vi "Load Config.vi"(8 "error in (no error)":errorcluster, 11 "Data Processor Module in":refnum<class "Data Processor Module.lvclass">) -> (0 "error out":errorcluster, 3 "Data Processor Module out":refnum<class "Data Processor Module.lvclass">)   [LabVIEW 2020, in "VolatusData.lvlib" / "Data Processor Module.lvclass"]
uses:
  Data Processor Module.lvclass
  Data Processor Module.lvclass/Data Processor Module.ctl
  Volatus/Module/Module.lvclass
  VolatusConfig/VolatusConfigElement/VolatusConfigElement.lvclass
  lv-cdm/CDM-Config/Config Element/Config Element.lvclass
  C:/dev/lv20CE/relink/lv-volatus/Volatus/Module/Module.lvclass
  C:/dev/lv20CE/relink/lv-volatus/VolatusData/Data Processor Module/Data Processor Module.lvclass
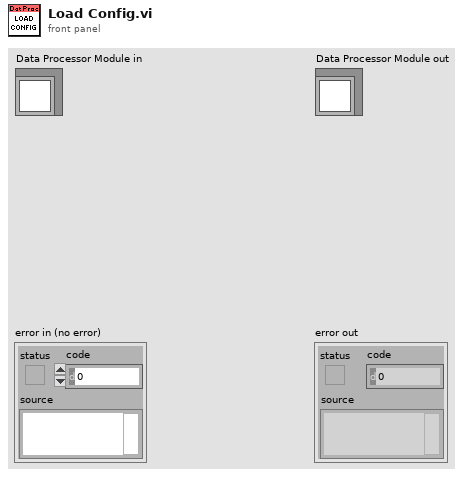
[diagram p1: front panel]
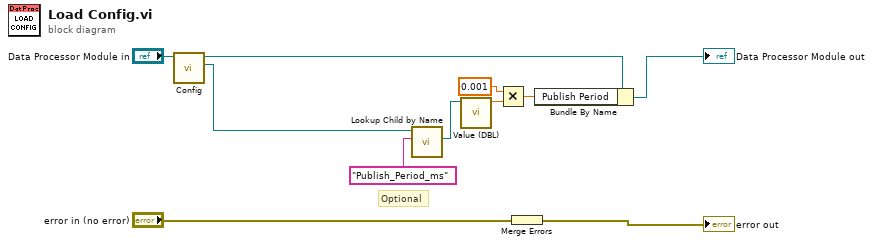
[diagram p0: block diagram]
diagram:
  # "Optional"
  n1 = call "Config.vi"("Module in"="Data Processor Module in") -> ("Config"=w8:refnum<class "VolatusConfigElement.lvclass">, "Module out"=w9:refnum<class "Data Processor Module.lvclass">)  [unwired: 9 in]
  n2 = call "Lookup Child by Name.vi"("Child Name"="Publish_Period_ms", "VolatusConfigElement in"=w8) -> ("Child"=w6:refnum<class "Config Element.lvclass">)  [unwired: 6 in, 3 out]
  n3 = call "Value (DBL).vi"("Config Element in"=w6) -> ("DBL Value"=w5:dbl)  [unwired: 9 in, 1 out]
  n4 = Multiply(x=0.001, y=w5) -> (x*y=w2:dbl)
  n5 = Merge Errors("error in (no error)") -> (→"error out":errorcluster)
  n6 = Bundle By Name(cluster=w9, "Publish Period"=w2) -> (→"Data Processor Module out":refnum<class "Data Processor Module.lvclass">)
